vi "Count Allocated Datums.vi"(1 "bytestream":refnum<class "Bytestream.lvclass">) -> (0 "datums":i32)   [LabVIEW 2020, in "NI_Bytestream.lvlib" / "Bytestream.lvclass"]
uses:
  <vilib>/Array/Bytestream/Bytestream.lvclass
  <vilib>/Array/Bytestream/Bytestream.lvclass/Bytestream.ctl
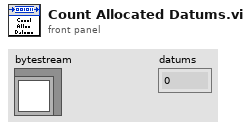
[diagram p1: front panel]
types:
  T1 = typedef "NI_Bytestream.lvlib/Bytestream.lvclass/Datum.ctl" = cluster{"array":u8[], "index":i32}
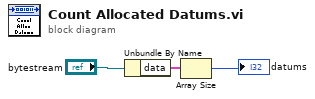
[diagram p0: block diagram]
diagram:
  n1 = Unbundle By Name("bytestream") -> ("data"=w2:T1[])
  n2 = Array Size(array=w2) -> (size(s)=→"datums":i32)
